vi "Log Messages.vi"(8 "error in (no error)":errorcluster, 10 "Actor to Log":refnum<class "Message Enqueuer.lvclass">, 11 "Monitor Window in":refnum<class "Classic Monitor.lvclass">) -> (0 "error out":errorcluster, 3 "Monitor Window out":refnum<class "Classic Monitor.lvclass">)   [LabVIEW 2017, in "MGI-Monitored Actor.lvlib" / "Classic Monitor.lvclass"]
doc: "Starts message logging on the specified actor\n\nCopyright: MGI 2016\nAuthor: Derek Trepanier"
uses:
  Classic Monitor.lvclass
  D:/software/LabView_MonitoredActor/monitored-actor-core/Source/Actor Monitor/Actor Monitor/Actor Monitor.lvclass
  C:/Program Files (x86)/National Instruments/LabVIEW 2017/vi.lib/ActorFramework/Actor/Actor.lvclass
  <vilib>/ActorFramework/Message Enqueuer/Message Enqueuer.lvclass
  monitored-actor-core/Source/Actor Monitor/Actor Monitor/Actor Monitor.lvclass/Actor Monitor.ctl
  Classic Monitor.lvclass/Classic Monitor.ctl
  Logger/Logger Actor/Classic Logger.lvclass
  Logger/Logger Messages/Start Logging Msg/Start Logging Msg.lvclass
  monitored-actor-core/Source/Actor Monitor/Actor Monitor/Actor Monitor.lvclass
  monitored-actor-core/Source/Monitor Data/Monitor Data.lvclass
  <vilib>/ActorFramework/Actor/Actor.lvclass
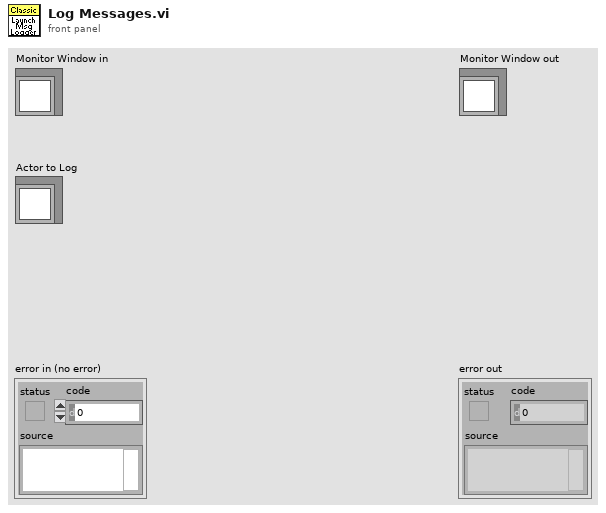
[diagram p1: front panel]
types:
  T1 = typedef "MGI-Monitored Actor Core.lvlib/Monitor Data.lvclass/Actor Data.ctl" = cluster{"Actor Type":string, "Actor Cores":string[], "Self":refnum<class "Message Enqueuer.lvclass">, "Caller":refnum<class "Message Enqueuer.lvclass">, "Actor Label":string, "Last Ping":dbl}
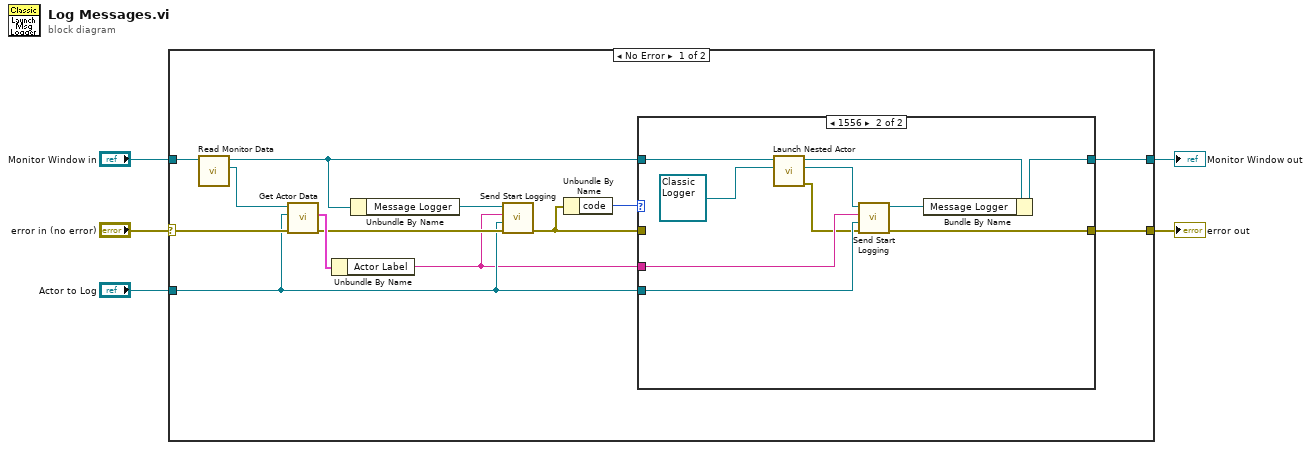
[diagram p0: block diagram]
diagram:
  n1 = case shown="No Error" "error in (no error)" {
    selector: "error in (no error)" -> [w15 w32]
    tunnel: [w16 w32] -> w4
    tunnel: [w18 w31] -> w2
    tunnel: "Monitor Window in" -> [w17 w31]
    tunnel: "Actor to Log" -> [w7 _]
    frame No Error {
      n2 = call "Read Monitor Data.vi"("Actor Monitor New in"=w17) -> ("Monitored Actor.lvlib:Monitor Data.lvclass"=w13:refnum<class "Monitor Data.lvclass">, "Actor Monitor New out"=w14:refnum<class "Classic Monitor.lvclass">)  [unwired: 8 in, 1 out]
      n3 = call "Get Actor Data.vi"("error in (no error)"=w15, "Actor's Self Q"=w7, "Monitor Data in"=w13) -> ("error out"=w9:errorcluster, "Actor Data"=w12:T1)  [unwired: 5 in, 2 out]
      n4 = Unbundle By Name(w12) -> ("Actor Label"=w6:string)
      n5 = Unbundle By Name(w14) -> ("Message Logger"=w10:refnum<class "Message Enqueuer.lvclass">)
      n6 = call "Send Start Logging.vi"("error in (no error)"=w9, "Actor to Log"=w7, "Label"=w6, "Message Enqueuer in"=w10) -> ("error out"=w8:errorcluster)  [unwired: 6 in, 1 out]
      n7 = Unbundle By Name(w8) -> ("code"=w11:i32)
      n8 = case shown="1556" w11 {
        tunnel: [w20 w30] -> w18
        tunnel: w14 -> [w20 w29]
        tunnel: w7 -> [_ w26]
        tunnel: w6 -> [_ w25]
        tunnel: [w19 w27] -> w16
        tunnel: w8 -> [w19 _]
        frame Default {
        }
        frame 1556 {
          n9 = call <vilib>:"Launch Nested Actor.vi"("Nested Actor"=refnum<class "Classic Logger.lvclass"> refnum ("Classic Monitor.lvlib:Message Logger.lvclass"), "Caller Actor in"=w29) -> ("error out"=w21:errorcluster, "Nested Actor's Enqueuer"=w23:refnum<class "Message Enqueuer.lvclass">, "Caller Actor in"=w24:refnum<class "Classic Monitor.lvclass">)  [unwired: 7 in]
          n10 = call "Send Start Logging.vi"("error in (no error)"=w21, "Actor to Log"=w26, "Label"=w25, "Message Enqueuer in"=w23) -> ("error out"=w27:errorcluster, "Message Enqueuer out"=w28:refnum<class "Message Enqueuer.lvclass">)  [unwired: 6 in]
          n11 = Bundle By Name(cluster=w24, "Message Logger"=w28) -> (w30:refnum<class "Classic Monitor.lvclass">)
        }
      }
    }
    frame Error {
    }
  }
  "error out" <- w4
  "Monitor Window out" <- w2
